vi "MainEnQueue.vi"(6 "Enqueue in Back?":bool, 8 "error in":errorcluster, 10 "Array States":T1[](array[typedef]), 11 "States":T1) -> (0 "error out":errorcluster)   [LabVIEW 2022 SP3]
uses:
  Type Def/MainStates Cluster.ctl
  Type Def/MainStates.ctl
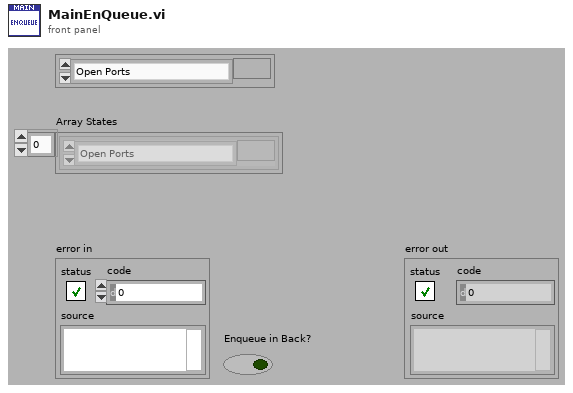
[diagram p1: front panel]
types:
  T1 = typedef "MainStates Cluster.ctl" = cluster{"States":T2, "Data":variant}
  T2 = typedef "MainStates.ctl" = enum16{"Open Ports", "Close Ports", "Main", "Settings", "Voltaje", "Probe", "Lenguaje", "Callibration", "Exit", "Voltage Test", "Test 2", "End test"}
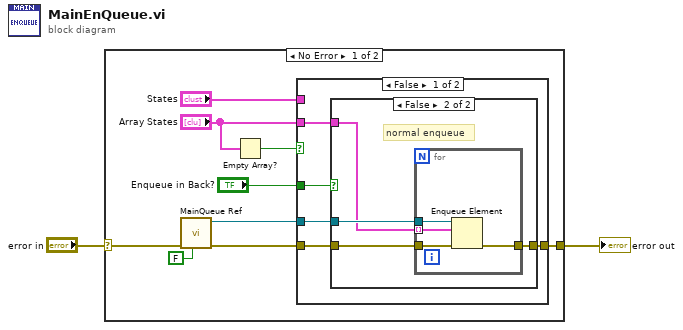
[diagram p0: block diagram]
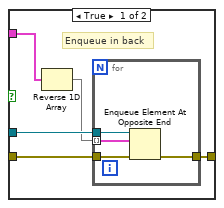
[diagram p2: hidden frame]
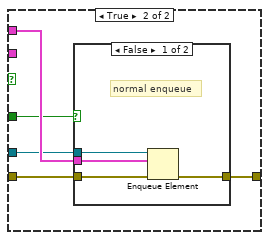
[diagram p3: hidden frame]
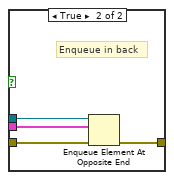
[diagram p4: hidden frame]
diagram:
  n1 = case shown="No Error" "error in" {
    selector: "error in" -> [w10 w47]
    tunnel: [w8 w47] -> w1
    frame No Error {
      n2 = call "MainQueue Ref.vi"("Write:T/Read:(F)"=FALSE ("Write:T/Read:F"), "error in"=w10) -> ("error out"=w9:errorcluster, "queue out"=w6:refnum<queue>)  [unwired: 8 in]
      n3 = Empty Array?(array="Array States") -> (empty?=w5:bool)
      n4 = case shown="False" w5 {
        tunnel: w9 -> [w15 w38]
        tunnel: [w14 w37] -> w8
        tunnel: "States" -> [_ w36]
        tunnel: w6 -> [w13 w35]
        tunnel: "Array States" -> [w16 _]
        tunnel: "Enqueue in Back?" -> [w12 w34]
        frame False {
          n5 = case shown="False" w12 {
            tunnel: w16 -> [w21 w26]
            tunnel: w15 -> [w20 w29]
            tunnel: [w19 w28] -> w14
            tunnel: w13 -> [w18 w27]
            frame True {
              # "Enqueue in back"
              n6 = Reverse 1D Array(array=w21) -> (reversed array=w17:T1[])
              n7 = for {
                tunnel: w20 -> [w25]
                tunnel: [w24] -> w19
                tunnel: w18 -> [w23]
                tunnel: w17 -> [w22] mode=indexing
                n8 = Enqueue Element At Opposite End(queue=w23, element=w22, error in (no error)=w25) -> (error out=w24:errorcluster)  [unwired: 1 in, 2 out]
              }
            }
            frame False {
              # "normal enqueue"
              n9 = for {
                tunnel: w29 -> [w33]
                tunnel: [w32] -> w28
                tunnel: w27 -> [w31]
                tunnel: w26 -> [w30] mode=indexing
                n10 = Enqueue Element(queue=w31, element=w30, error in (no error)=w33) -> (error out=w32:errorcluster)  [unwired: 1 in, 2 out]
              }
            }
          }
        }
        frame True {
          n11 = case shown="False" w34 {
            tunnel: w38 -> [w42 w46]
            tunnel: [w41 w45] -> w37
            tunnel: w36 -> [w40 w43]
            tunnel: w35 -> [w39 w44]
            frame False {
              # "normal enqueue"
              n12 = Enqueue Element(queue=w39, element=w40, error in (no error)=w42) -> (error out=w41:errorcluster)  [unwired: 1 in, 2 out]
            }
            frame True {
              # "Enqueue in back"
              n13 = Enqueue Element At Opposite End(queue=w44, element=w43, error in (no error)=w46) -> (error out=w45:errorcluster)  [unwired: 1 in, 2 out]
            }
          }
        }
      }
    }
    frame Error {
    }
  }
  "error out" <- w1
